vi "2023_day13 (SubVI Search in Rows and Cols).vi"(7 "Ignore Case":i32[](array[numeric])=[-1, -1], 11 "Character Array":string[][](array[string])) -> (1 "Match Index":i32, 2 "Match Found?":bool, 3 "Row or Col":enum32{"Row", "Col"}(ring))   [LabVIEW 2021]
uses:
  <userlib>/_OpenG.lib/array/array.llb/Reverse 2D Array (String)__ogtk.vi
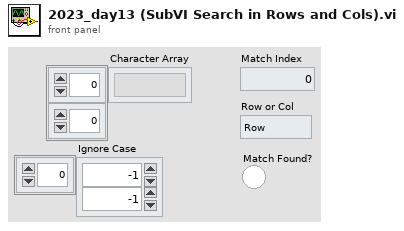
[diagram p1: front panel]
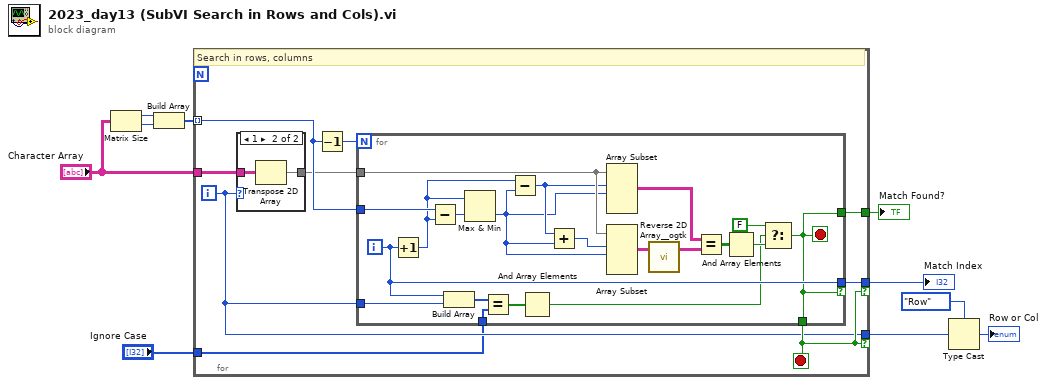
[diagram p0: block diagram]
diagram:
  n1 = Matrix Size(0:"Character Array") -> (1:w6:i32, 2:w7:i32)
  n2 = Build Array(w6, w7) -> (w8:i32[])
  n3 = for {
    tunnel: w8 -> [w18] mode=indexing
    tunnel: "Character Array" -> [w16]
    tunnel: [w12] -> w10 if=w14
    tunnel: [w15] -> w9 if=w14
    tunnel: [w13] -> w3
    tunnel: "Ignore Case" -> [w11]
    i -> [w12]
    stop <- w14 stop-if-true
    # "Search in rows, columns"
    n4 = case shown="1" w12 {
      tunnel: [w20 w21] -> w17
      tunnel: w16 -> [w20 w22]
      frame 0, Default {
      }
      frame 1 {
        n5 = Transpose 2D Array(2D array=w22) -> (transposed array=w21:string[][])
      }
    }
    n6 = Decrement(x=w18) -> (x-1=w19:i32)
    n7 = for {
      N: w19 -> [_]
      tunnel: w17 -> [w39]
      tunnel: w18 -> [w42]
      tunnel: [w31] -> w15 if=w30
      tunnel: [w30] -> w14
      tunnel: [w30] -> w13
      tunnel: w12 -> [w32]
      tunnel: w11 -> [w26]
      i -> [w31]
      stop <- w30 stop-if-true
      n8 = Increment(x=w31) -> (x+1=w40:i32)
      n9 = Subtract(x=w42, y=w40) -> (x-y=w41:i32)
      n10 = Build Array(w31, w32) -> (w27:i32[])
      n11 = Max & Min(x=w40, y=w41) -> (min(x,y)=w37:i32)  [unwired: 1 out]
      n12 = Equal?(x=w27, y=w26) -> (x = y?=w25:bool[])
      n13 = Subtract(x=w40, y=w37) -> (x-y=w38:i32)
      n14 = And Array Elements(Boolean array=w25) -> (logical AND=w24:bool)
      n15 = Add(x=w38, y=w37) -> (x+y=w36:i32)
      n16 = Array Subset(array=w39, index (row)=w38, length (row)=w37) -> (w33:string[][])  [unwired: 2 in]
      n17 = Array Subset(array=w39, index (row)=w36, length (row)=w37) -> (w35:string[][])  [unwired: 2 in]
      n18 = call-poly <userlib>:"Reverse 2D Array__ogtk.vi"("Array"=w35) -> ("Reversed Array"=w23:string[][])  [unwired: 2 in]
      n19 = Equal?(x=w33, y=w23) -> (x = y?=w34:bool[][])
      n20 = And Array Elements(Boolean array=w34) -> (logical AND=w29:bool)
      n21 = Select(t=FALSE, s=w24, f=w29) -> (s? t:f=w30:bool)
    }
  }
  "Match Index" <- w9
  "Match Found?" <- w3
  n22 = Type Cast(type=enum32{"Row", "Col"}."Row", x=w10) -> (*(type *) &x=→"Row or Col":enum32{"Row", "Col"})
